vi "TitleData_GRR.vi"(8 "error in (no error)":errorcluster caption="错误输入（无错误）", 10 "Tabledata in":string[][](array[string]), 11 "Step":enum16{"Initial", "Write", "Read"}(ring)) -> (0 "error out":errorcluster caption="错误输出", 3 "Tabledata Out":string[][](array[string]))   [LabVIEW 2017]
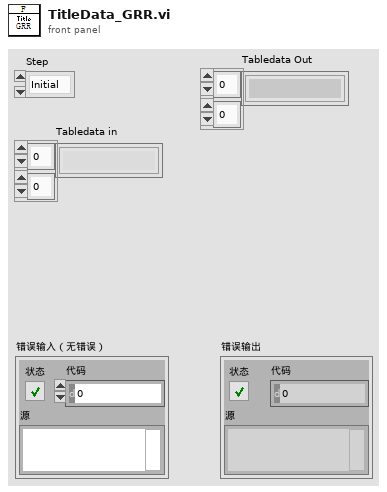
[diagram p1: front panel]
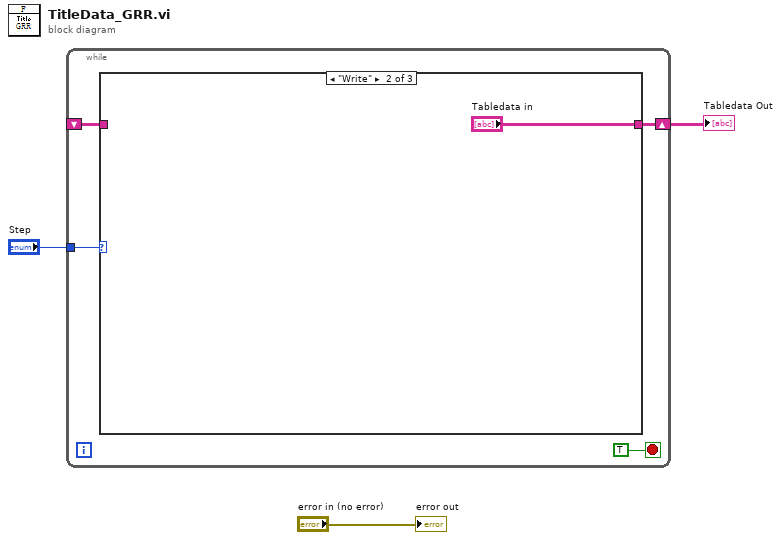
[diagram p0: block diagram]
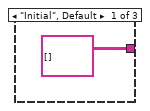
[diagram p2: hidden frame]
diagram:
  n1 = while {
    tunnel: "Step" -> [w7]
    shift-right: [w5] -> w1
    shift-left: _ -> [w4]
    stop <- TRUE stop-if-true
    n2 = case shown="\"Write\"" w7 {
      tunnel: [string[][] [] ("DIConfigIn") "Tabledata in" w10] -> w5
      tunnel: w4 -> [_ _ w10]
      frame "Initial", Default {
      }
      frame "Write" {
      }
      frame "Read" {
      }
    }
  }
  "Tabledata Out" <- w1
  "error out" <- "error in (no error)"
